vi "fpga_project.vi"() -> ()   [LabVIEW 2019]
uses:
  <vilib>/Platform/TimedLoop/XDataNode/timing_clust.ctl
  <vilib>/Platform/TimedLoop/XDataNode/nitl_modes.ctl
  <vilib>/Platform/TimedLoop/XDataNode/wakeup.ctl
  <vilib>/rvi/Emulation/niFpgaGetClockAttributes.vi
  <vilib>/rvi/Emulation/niFpgaSctlEmulationGetInTimedLoop.vi
  <vilib>/rvi/Emulation/niFpgaEmulationReportErrorSimple.vi
  <vilib>/rvi/eio/common/nirviEmuTemplateMethod_errors.vi
  <vilib>/rvi/Emulation/niFpgaCriticalErrorInLSC.vi
  <vilib>/eio/EIONode/EIONode.xnode
  <vilib>/eio/EIOMethodNode/EIOMethodNode.xnode
  <vilib>/platform/TimedLoop/XDataNode/XDataNode.xnode
  <vilib>/Platform/TimedLoop/XDataNode/XDNodeRunTimeDep.lvlib
panel:
  out "Array 2":bool[](array[boolean])
  out "Array":bool[](array[boolean])
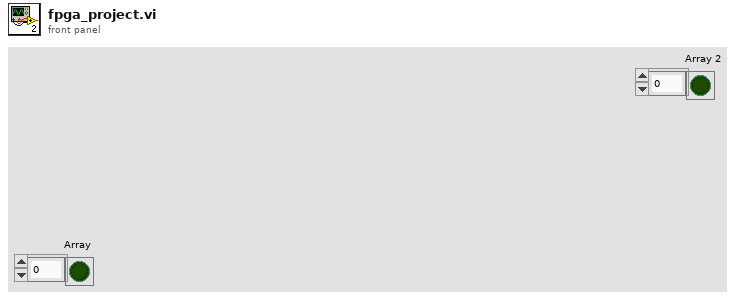
[diagram p1: front panel]
types:
  T1 = typedef "XDNodeRunTimeDep.lvlib/timing_clust.ctl" = cluster{"Expected End [f-1]":u64, "Actual End [f-1]":u64, "Finished Late? [f-1]":bool, "Expected End [i-1]":u64, "Actual End [i-1]":u64, "Finished Late? [i-1]":bool, "Expected Start [i]":u64, "Actual Start [i]":u64, "Expected Start [f]":u64, "Actual Start [f]":u64, "Source Name":string, "Structure Name":string, "Period":i64, "Deadline":i64, "Offset":i64, "Start":i64, "Priority":i32, "Timeout":i32, "Mode":T2, "Wakeup Reason":T3, "Error":errorcluster, "Source Type":string, "Secondary Source Type":string, "Global End Time":u64, "Global Start Time":u64, "Frame Duration":u64, "Iteration Duration":u64, "Assigned CPU":i32, "I/O Scan Engine Mode":u32}
  T2 = typedef "XDNodeRunTimeDep.lvlib/nitl_modes.ctl" = enum32{"No Change", "Process missed periods, maintain original phase", "Discard missed periods, maintain original phase", "Process missed periods, ignore original phase", "Discard missed periods, ignore original phase"}
  T3 = typedef "XDNodeRunTimeDep.lvlib/wakeup.ctl" = enum32{"Normal", "Aborted", "Asynchronous wakeup", "Timing source error", "Timed loop error", "Timeout"}
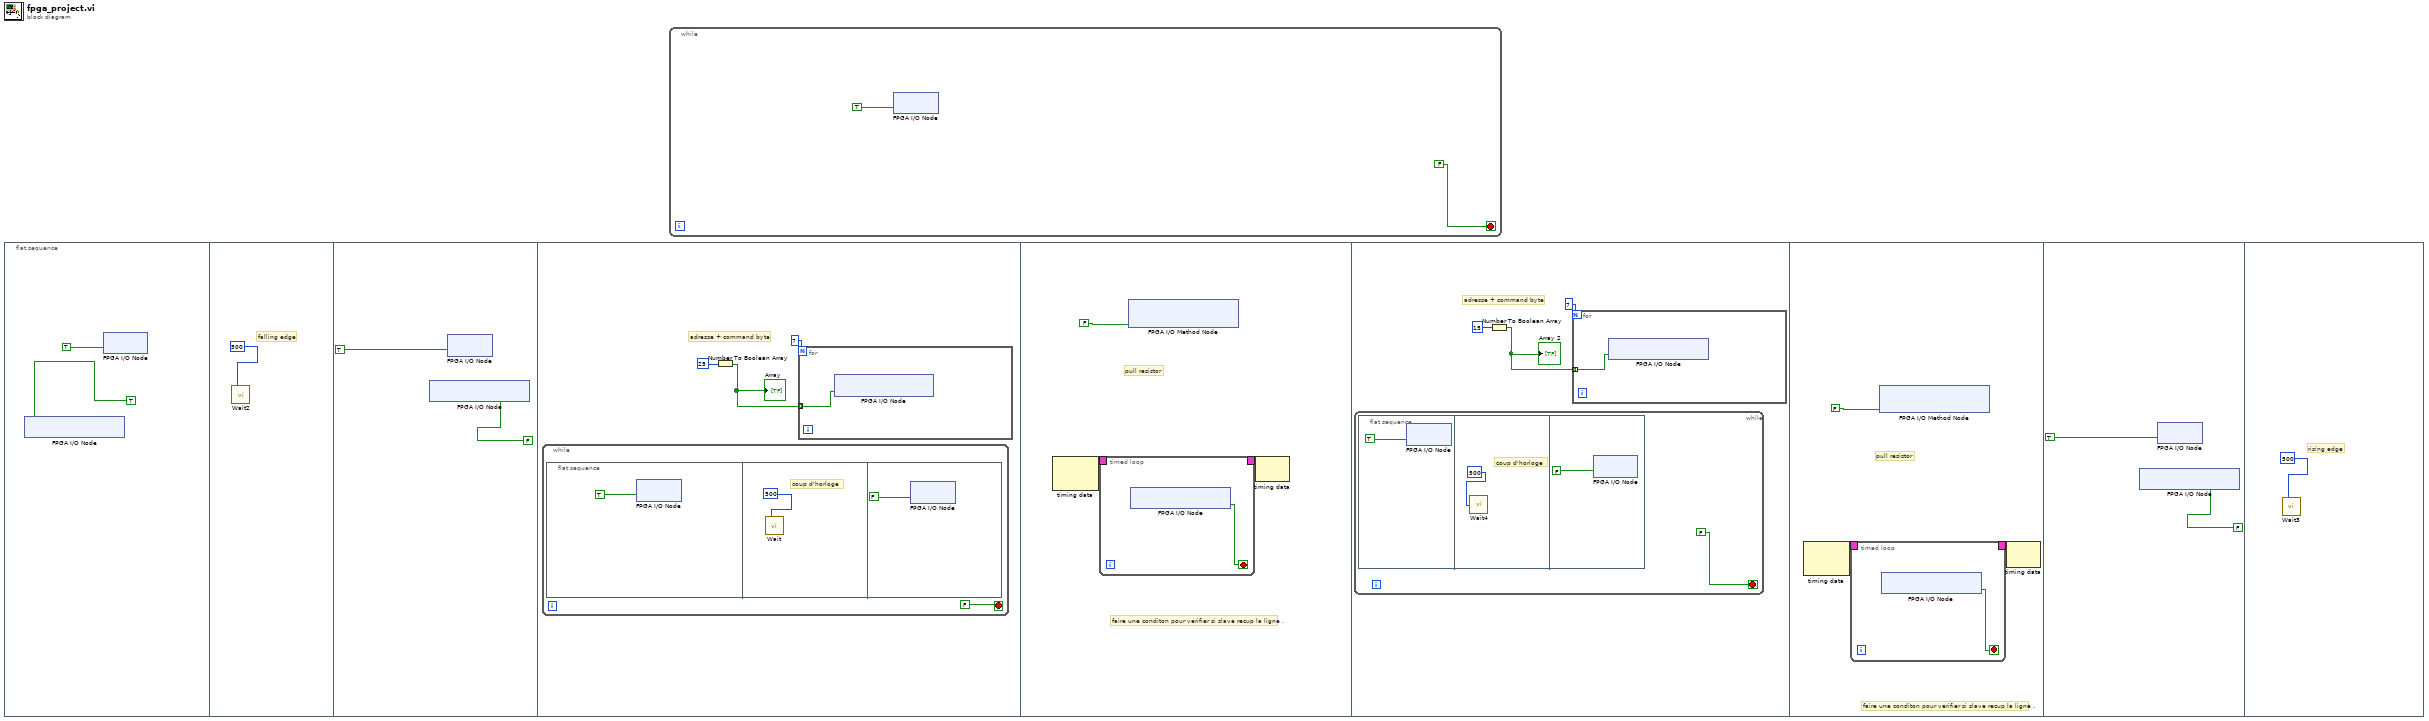
[diagram p0: block diagram]
diagram:
  n1 = flat-sequence {
    frame #0 {
      n2 = xnode "FPGA I/O Node"("ConnectorB/DIO15  SDA"=TRUE) -> ()  [unwired: 1 in, 1 out]
      n3 = xnode "FPGA I/O Node"("CLK"=TRUE) -> ()  [unwired: 1 in, 1 out]
    }
    frame #1 {
      # "falling edge"
      n4 = call "Wait2"("Count(Ticks)"=u32 500) -> ()  [unwired: 1 out]
    }
    frame #2 {
      n5 = xnode "FPGA I/O Node"("ConnectorB/DIO15  SDA"=FALSE) -> ()  [unwired: 1 in, 1 out]
      n6 = xnode "FPGA I/O Node"("CLK"=TRUE) -> ()  [unwired: 1 in, 1 out]
    }
    frame #3 {
      # "adresse + command byte"
      n7 = while {
        stop <- FALSE stop-if-true
        n8 = flat-sequence {
          frame #0 {
            n9 = xnode "FPGA I/O Node"("CLK"=TRUE) -> ()  [unwired: 1 in, 1 out]
          }
          frame #1 {
            # "coup d'horloge"
            n10 = call "Wait"("Count(Ticks)"=u32 500) -> ()  [unwired: 1 out]
          }
          frame #2 {
            n11 = xnode "FPGA I/O Node"("CLK"=FALSE) -> ()  [unwired: 1 in, 1 out]
          }
        }
      }
      n12 = Number To Boolean Array(number=u8 25) -> (Boolean array=w7:bool[])
      "Array" <- w7
      n13 = for {
        N: 7 -> [_]
        tunnel: w7 -> [w13] mode=indexing
        n14 = xnode "FPGA I/O Node"("ConnectorB/DIO15  SDA"=w13) -> ()  [unwired: 1 in, 1 out]
      }
    }
    frame #4 {
      # "faire une conditon pour verifier si slave recup la ligne ."
      # "pull resistor"
      n15 = node-c288() -> (w15:T1)  [unwired: 2 in]
      n16 = timed-loop {
        timing: w15 -> [_]
        timing-out: [_] -> w14
        stop <- w17 stop-if-true
        n17 = xnode "FPGA I/O Node"() -> ("ConnectorB/DIO15  SDA"=w17:bool)  [unwired: 1 in, 1 out]
      }
      n18 = xnode "FPGA I/O Method Node"("Enable"=FALSE) -> ()  [unwired: 1 in, 1 out]
      n19 = node-c288(w14) -> ()  [unwired: 1 out]
    }
    frame #5 {
      # "adresse + command byte"
      n20 = while {
        stop <- FALSE stop-if-true
        n21 = flat-sequence {
          frame #0 {
            n22 = xnode "FPGA I/O Node"("CLK"=TRUE) -> ()  [unwired: 1 in, 1 out]
          }
          frame #1 {
            # "coup d'horloge"
            n23 = call "Wait4"("Count(Ticks)"=u32 500) -> ()  [unwired: 1 out]
          }
          frame #2 {
            n24 = xnode "FPGA I/O Node"("CLK"=FALSE) -> ()  [unwired: 1 in, 1 out]
          }
        }
      }
      n25 = Number To Boolean Array(number=u8 15) -> (Boolean array=w23:bool[])
      "Array 2" <- w23
      n26 = for {
        N: 7 -> [_]
        tunnel: w23 -> [w29] mode=indexing
        n27 = xnode "FPGA I/O Node"("ConnectorB/DIO15  SDA"=w29) -> ()  [unwired: 1 in, 1 out]
      }
    }
    frame #6 {
      # "faire une conditon pour verifier si slave recup la ligne ."
      # "pull resistor"
      n28 = node-c288() -> (w32:T1)  [unwired: 2 in]
      n29 = timed-loop {
        timing: w32 -> [_]
        timing-out: [_] -> w31
        stop <- w33 stop-if-true
        n30 = xnode "FPGA I/O Node"() -> ("ConnectorB/DIO15  SDA"=w33:bool)  [unwired: 1 in, 1 out]
      }
      n31 = xnode "FPGA I/O Method Node"("Enable"=FALSE) -> ()  [unwired: 1 in, 1 out]
      n32 = node-c288(w31) -> ()  [unwired: 1 out]
    }
    frame #7 {
      n33 = xnode "FPGA I/O Node"("ConnectorB/DIO15  SDA"=FALSE) -> ()  [unwired: 1 in, 1 out]
      n34 = xnode "FPGA I/O Node"("CLK"=TRUE) -> ()  [unwired: 1 in, 1 out]
    }
    frame #8 {
      # "rising edge"
      n35 = call "Wait3"("Count(Ticks)"=u32 500) -> ()  [unwired: 1 out]
    }
  }
  n36 = while {
    stop <- FALSE stop-if-true
    n37 = xnode "FPGA I/O Node"("CLK"=TRUE) -> ()  [unwired: 1 in, 1 out]
  }
